vi "dashboardNames.vi"() -> (0 "String Names":string[](array[string])=["DB/Button 0", "DB/Button 1", "DB/Button 2", "DB/Button 3"], 1 "Slider Names":string[](array[string])=["DB/Button 0", "DB/Button 1", "DB/Button 2", "DB/Button 3"], 2 "LED Names":string[](array[string])=["DB/Button 0", "DB/Button 1", "DB/Button 2", "DB/Button 3"], 3 "Button Names":string[](array[string])=["DB/Button 0", "DB/Button 1", "DB/Button 2", "DB/Button 3"])   [LabVIEW 2016]
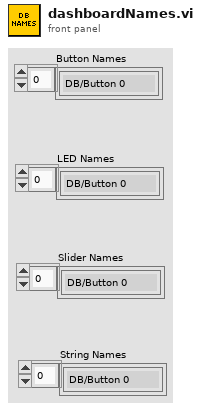
[diagram p1: front panel]
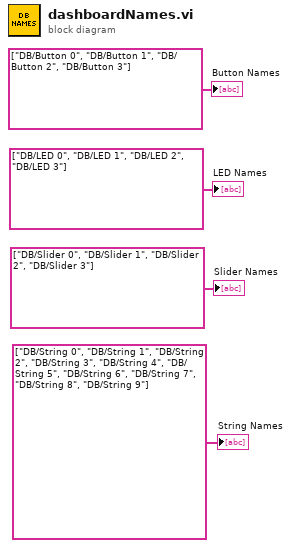
[diagram p0: block diagram]
diagram:
  "Button Names" <- string[] ["DB/Button 0", "DB/Button 1", "DB/Button 2", "DB/Button 3"]
  "LED Names" <- string[] ["DB/LED 0", "DB/LED 1", "DB/LED 2", "DB/LED 3"]
  "Slider Names" <- string[] ["DB/Slider 0", "DB/Slider 1", "DB/Slider 2", "DB/Slider 3"]
  "String Names" <- string[] ["DB/String 0", "DB/String 1", "DB/String 2", "DB/String 3", "DB/String 4", "DB/String 5", "DB/String 6", "DB/String 7", "DB/String 8", "DB/String 9"]
